vi "Restart DAQ.vi"(5 "Min Value":dbl, 6 "tiempo (s)":dbl, 7 "Max Value":dbl, 8 "error IN":errorcluster, 9 "Fs (S/s)":dbl, 10 "Physical Channel":tag, 11 "task IN":refnum<k21>) -> (0 "error OUT":errorcluster, 2 "# samples":u32, 3 "task OUT":refnum<k21>)   [LabVIEW 2010]
uses:
  <vilib>/Utility/error.llb/DialogType.ctl
  <vilib>/DAQmx/create/channels.llb/DAQmx Create Channel (AO-Voltage-Basic).vi
  <vilib>/DAQmx/configure/timing.llb/DAQmx Timing (Use Waveform).vi
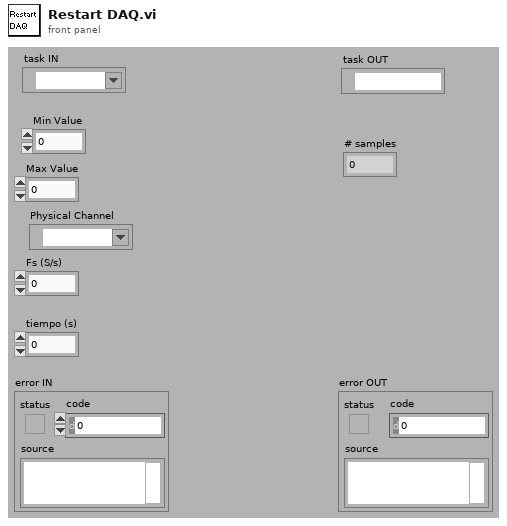
[diagram p1: front panel]
types:
  T1 = typedef "DialogType.ctl" = u16
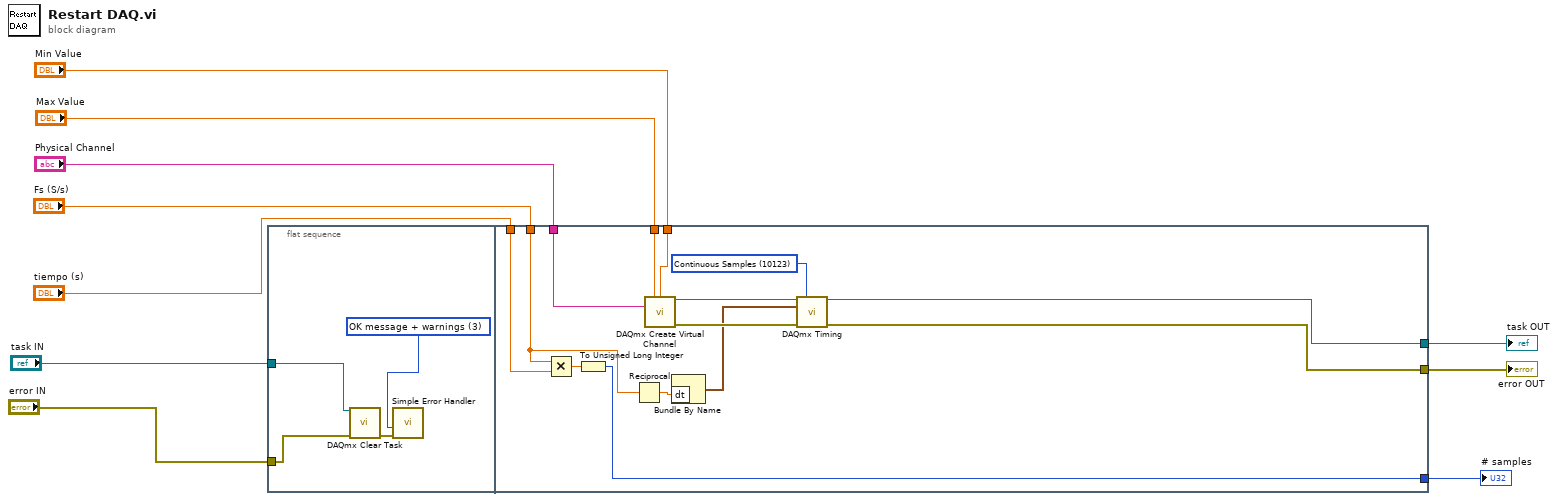
[diagram p0: block diagram]
diagram:
  n1 = flat-sequence {
    tunnel: "error IN" -> [w11]
    tunnel: "task IN" -> [w12]
    tunnel: [w28] -> w10
    tunnel: [w27] -> w9
    tunnel: [w26] -> w8
    tunnel: "Physical Channel" -> [w19]
    tunnel: "tiempo (s)" -> [w18]
    tunnel: "Fs (S/s)" -> [w15]
    tunnel: "Max Value" -> [w17]
    tunnel: "Min Value" -> [w16]
    frame #0 {
      w14 = T1 3 items=["no dialog", "OK message", "continue or stop message", "OK message + warnings", "continue/stop + warnings"] ("type of dialog (OK msg:1)")
      n2 = call <vilib>:"DAQmx Clear Task.vi"("task in"=w12, "error in"=w11) -> ("error out"=w13:errorcluster)  [unwired: 13 in]
      n3 = call <vilib>:"Simple Error Handler.vi"("type of dialog (OK msg:1)"=w14, "error in (no error)"=w13) -> ()  [unwired: 3 in, 5 out]
    }
    frame #1 {
      w21 = 10123 items=["Finite Samples"=10178, "Continuous Samples"=10123, "Hardware Timed Single Point"=12522] ("sample mode")
      n4 = Multiply(x=w15, y=w18) -> (x*y=w20:dbl)
      n5 = To Unsigned Long Integer(number=w20) -> (unsigned 32bit integer=w26:u32)
      n6 = Reciprocal(x=w15) -> (1/x=w25:dbl)
      n7 = call-poly <vilib>:"DAQmx Create Virtual Channel.vi"("maximum value"=w17, "minimum value"=w16, "physical channels"=w19) -> ("task out"=w23:refnum<k21>, "error out"=w24:errorcluster)  [unwired: 11 in]
      n8 = Bundle By Name("dt"=w25) -> (w22:waveform(dbl))  [unwired: 1 in]
      n9 = call-poly <vilib>:"DAQmx Timing.vi"("task/channels in"=w23, "sample mode"=w21, "waveform"=w22, "error in"=w24) -> ("task out"=w28:refnum<k21>, "error out"=w27:errorcluster)  [unwired: 10 in]
    }
  }
  "task OUT" <- w10
  "error OUT" <- w9
  "# samples" <- w8
